vi "readMagnetInfo.vi"(8 "error in (no error)":errorcluster) -> (0 "DS read error":errorcluster, 3 "output cluster":T1={"Main interlock"=TRUE, "Flow Switch 1"=TRUE, "Flow Switch 2"=TRUE, "Power Supply ok"=FALSE, "on"=TRUE, "staging"=TRUE, "undulator"=FALSE, "VOLTAGE"=0.0, "CURRENT"=0.0, "curent set"=0})   [LabVIEW 2013]
uses:
  MagnetCluster.ctl
panel:
  out "curent set":u16
  out "CURRENT":dbl
  out "VOLTAGE":dbl
  out "undulator":bool
  out "staging":bool
  out "on":bool
  out "Power Supply ok":bool
  out "Flow Switch 2":bool
  out "Flow Switch 1":bool
  out "Main interlock":bool
  out "Boolean array":bool[](array[boolean])
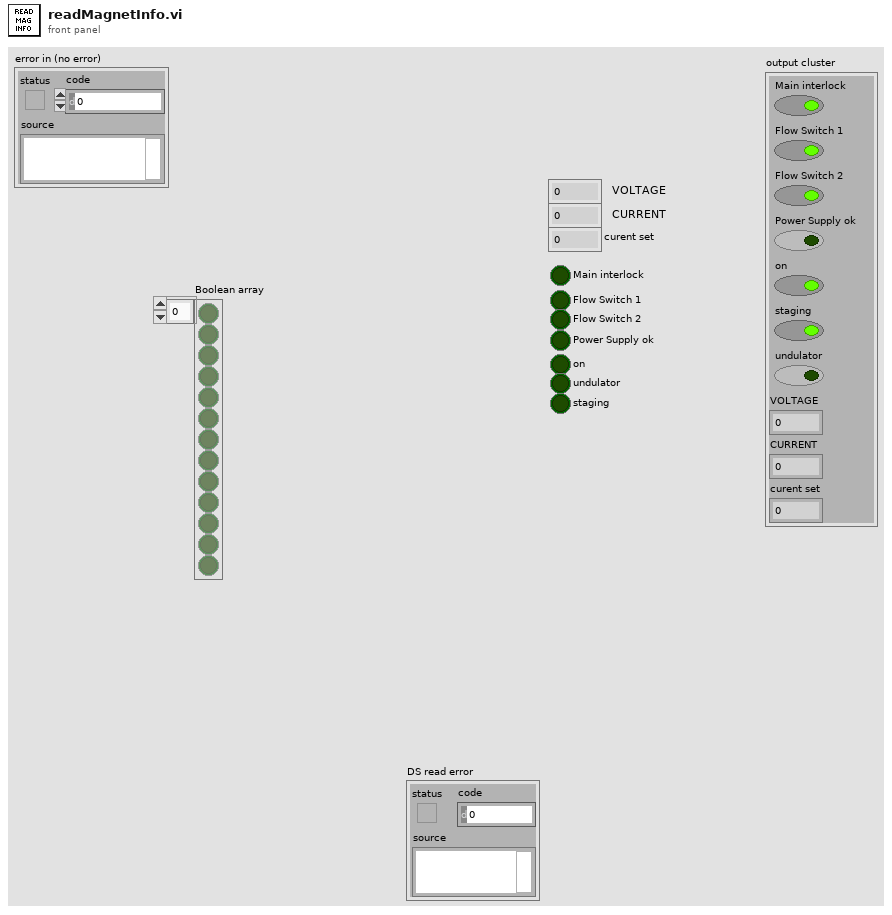
[diagram p1: front panel]
types:
  T1 = typedef "MagnetCluster.ctl" = cluster{"Main interlock":bool, "Flow Switch 1":bool, "Flow Switch 2":bool, "Power Supply ok":bool, "on":bool, "staging":bool, "undulator":bool, "VOLTAGE":dbl, "CURRENT":dbl, "curent set":u16}
  T2 = cluster{string, string, string, string, string, string, string, string, string, string, string, string}
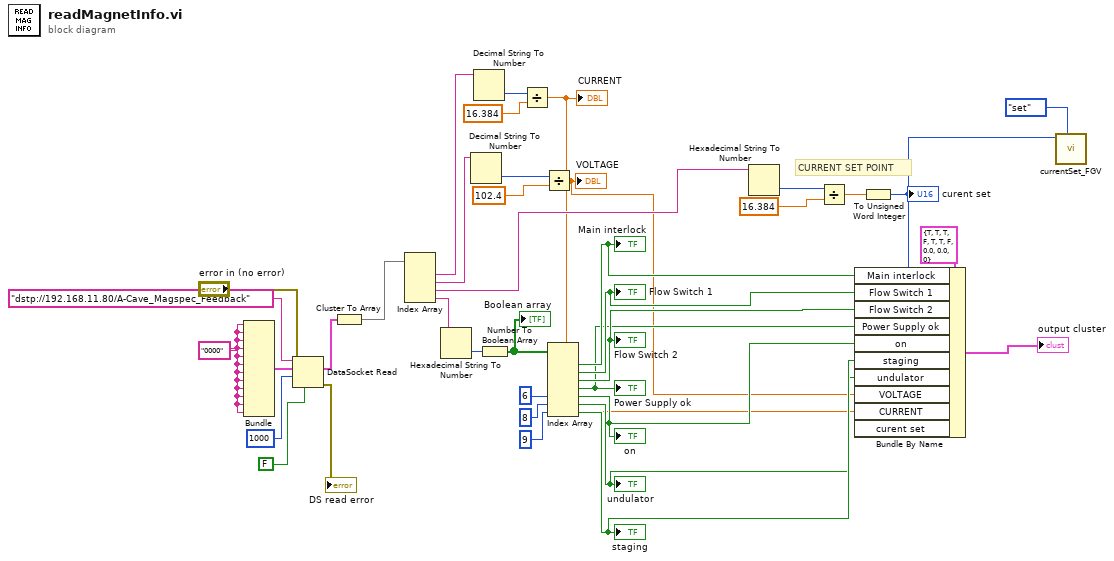
[diagram p0: block diagram]
diagram:
  w36 = "0000"
  # "CURRENT SET POINT"
  n1 = Bundle(w36, w36, w36, w36, w36, w36, w36, w36, w36, w36, w36, w36) -> (w33:T2)  [unwired: 1 in]
  n2 = DataSocket Read(6:FALSE ("wait for updated value (T)"), 8:"error in (no error)", 9:1000 ("ms timeout (10000)"), 10:w33, 11:"dstp://192.168.11.80/A-Cave_Magspec_Feedback" ("Source_URL")) -> (0:→"DS read error":errorcluster, 2:w32:T2)  [unwired: 5 out]
  n3 = Cluster To Array(cluster=w32) -> (array=w31:string[])
  n4 = Index Array(array=w31) -> (element #1=w21:string, element #2=w20:string, element #3=w15:string, element #4=w19:string)  [unwired: 4 in]
  n5 = Hexadecimal String To Number(string=w19) -> (number=w30:u32)  [unwired: 2 in, 1 out]
  n6 = Decimal String To Number(string=w20) -> (number=w24:i32)  [unwired: 2 in, 1 out]
  n7 = Decimal String To Number(string=w21) -> (number=w23:i32)  [unwired: 2 in, 1 out]
  n8 = Number To Boolean Array(number=w30) -> (Boolean array=w29:bool[])
  "Boolean array" <- w29
  n9 = Divide(x=w23, y=16.384) -> (x/y=w5:dbl)
  "CURRENT" <- w5
  n10 = Divide(x=w24, y=102.4) -> (x/y=w6:dbl)
  "VOLTAGE" <- w6
  n11 = Index Array(array=w29, index #5=6 ("index"), index #6=8 ("index"), index #7=9 ("index")) -> (element #1=w13:bool, element #2=w12:bool, element #3=w11:bool, element #4=w10:bool, element #5=w9:bool, element #6=w7:bool, element #7=w8:bool)  [unwired: 4 in]
  "Main interlock" <- w13
  "Flow Switch 1" <- w12
  "Flow Switch 2" <- w11
  "Power Supply ok" <- w10
  "on" <- w9
  "staging" <- w8
  "undulator" <- w7
  n12 = Hexadecimal String To Number(string=w15) -> (number=w17:u32)  [unwired: 2 in, 1 out]
  n13 = Divide(x=w17, y=16.384) -> (x/y=w18:dbl)
  n14 = To Unsigned Word Integer(number=w18) -> (unsigned 16bit integer=w3:u16)
  "curent set" <- w3
  n15 = Bundle By Name(cluster=T1 {"Main interlock"=TRUE, "Flow Switch 1"=TRUE, "Flow Switch 2"=TRUE, "Power Supply ok"=FALSE, "on"=TRUE, "staging"=TRUE, "undulator"=FALSE, "VOLTAGE"=0.0, "CURRENT"=0.0, "curent set"=0} ("Cluster"), "Main interlock"=w13, "Flow Switch 1"=w12, "Flow Switch 2"=w11, "Power Supply ok"=w10, "on"=w9, "staging"=w8, "undulator"=w7, "VOLTAGE"=w6, "CURRENT"=w5, "curent set"=w3) -> (→"output cluster":T1)
  n16 = call "currentSet_FGV.vi"("Enum"=enum16{"set", "read"}."set", "curent set"=w3) -> ()  [unwired: 9 in, 1 out]
